vi "Set_BSA_voltage_On_Off.vi"(0 "GPIB address":string, 2 "High Voltage":bool, 3 "error in (no error)":errorcluster) -> (7 "error out":errorcluster)   [LabVIEW 2010]
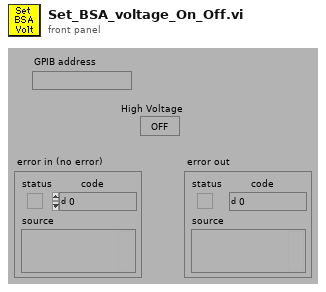
[diagram p1: front panel]
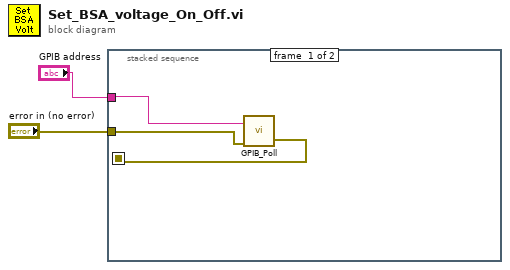
[diagram p0: block diagram]
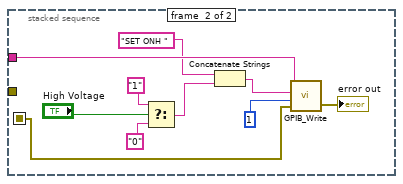
[diagram p2: hidden frame]
diagram:
  n1 = stacked-sequence {
    seq-local: [w3 _] -> [_ w14]
    tunnel: "GPIB address" -> [w5 w15]
    tunnel: "error in (no error)" -> [w4 _]
    frame #0 {
      n2 = call "GPIB_Poll.vi"("error in"=w4, "address string"=w5) -> ("error out"=w3:errorcluster)  [unwired: 1 out]
    }
    frame #1 {
      n3 = Select(t="1", s="High Voltage", f="0") -> (s? t:f=w8:string)
      n4 = Concatenate Strings("SET ONH ", w8) -> (w7:string)
      n5 = call "GPIB_Write.vi"("address string"=w15, "data In"=w7, "mode (0)"=i16 1, "error in"=w14) -> ("error out"=→"error out":errorcluster)  [unwired: 1 in, 1 out]
    }
  }
